vi "Timestamps_global.vi"() -> ()   [LabVIEW 2021]
panel:
  in  "Elution Timestamp":string="2023-07-19 15:29:12"
  in  "Sampling Timestamp":string="2023-07-19 15:23:13"
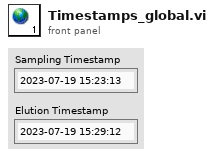
[diagram p1: front panel]
diagram:
